vi "configAO_phi.vi"(7 "address":string, 8 "error in (no error)":errorcluster, 9 "new phi (deg)":dbl, 10 "AO Channel":i32, 11 "Channels: AO":T1={"AO amp (V)"=[0.01, 0.0, 0.0, 0.0, 0.0, 0.0, 0.0, 0.0], "AO DC (V)"=[0.0, 0.0, 0.0, 0.0, 0.0, 0.0, 0.0, 0.0], "AO f (Hz)"=[13.1, 13.0, 13.0, 13.0, 13.0, 13.0, 13.0, 13.0], "AO phi (deg)"=[0.0, 0.0, 0.0, 0.0, 0.0, 0.0, 0.0, 0.0], "function"=[enum."Sine Wave", enum."Sine Wave", enum."Sine Wave", enum."Sine Wave", enum."Sine Wave", enum."Sine Wave", enum."Sine Wave", enum."Sine Wave"]} {"AO f (Hz)" min=0.001 max=10000.0; "AO DC (V)" format="%#_6p"; "AO amp (V)" format="%#_6p"}) -> (0 "error out":errorcluster, 3 "Channels: AO":T1={"AO amp (V)"=[0.01, 0.0, 0.0, 0.0, 0.0, 0.0, 0.0, 0.0], "AO DC (V)"=[0.0, 0.0, 0.0, 0.0, 0.0, 0.0, 0.0, 0.0], "AO f (Hz)"=[13.1, 13.0, 13.0, 13.0, 13.0, 13.0, 13.0, 13.0], "AO phi (deg)"=[0.0, 0.0, 0.0, 0.0, 0.0, 0.0, 0.0, 0.0], "function"=[enum."Sine Wave", enum."Sine Wave", enum."Sine Wave", enum."Sine Wave", enum."Sine Wave", enum."Sine Wave", enum."Sine Wave", enum."Sine Wave"]} {"AO f (Hz)" min=0.001 max=10000.0; "AO DC (V)" format="%#_6p"; "AO amp (V)" format="%#_6p"})   [LabVIEW 2016]
doc: "API to configure an AO phase.\n\nSpecify which channel you want to change and the value you want to set.\n\nIf address=\"\", this API reads from localhost\nIf address is remote lockin, you need to add this computer to allowed whitelist on the lockin computer you are trying to access."
uses:
  Typedefs/AO-cluster.ctl
  Typedefs/AO_Amp-array.ctl
  Typedefs/AO_DC-array.ctl
  Typedefs/AO_f-array.ctl
  Typedefs/AO_phi-array.ctl
  Typedefs/Function-array.ctl
  Typedefs/Function-enum.ctl
panel:
  # "0"
  # "1"
  # "2"
  # "3"
  # "4"
  # "5"
  # "6"
  # "7"
  # "0"
  # "1"
  # "2"
  # "3"
  # "4"
  # "5"
  # "6"
  # "7"
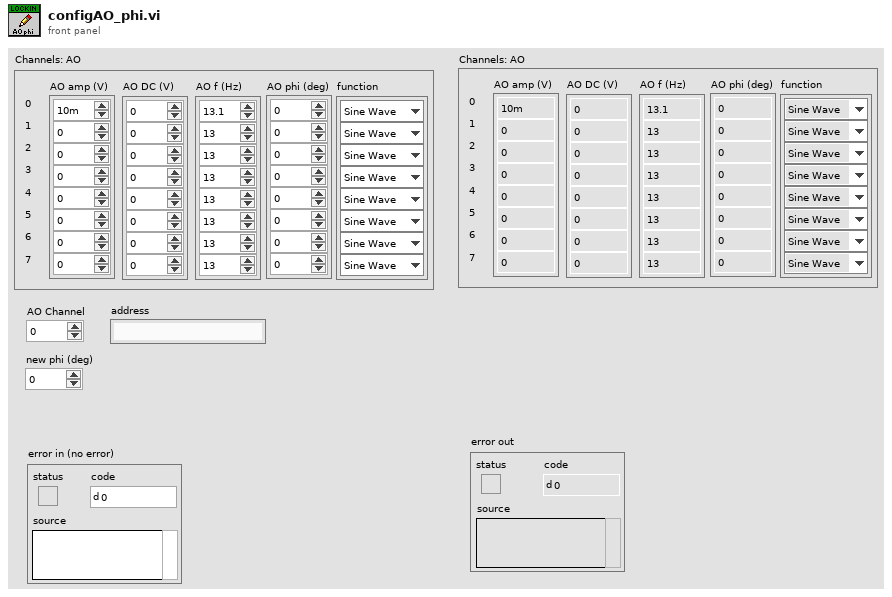
[diagram p1: front panel]
types:
  T1 = typedef "AO-cluster.ctl" = cluster{"AO amp (V)":T2, "AO DC (V)":T3, "AO f (Hz)":T4, "AO phi (deg)":T5, "function":T6}
  T2 = typedef "AO_Amp-array.ctl" = dbl[]
  T3 = typedef "AO_DC-array.ctl" = dbl[]
  T4 = typedef "AO_f-array.ctl" = dbl[]
  T5 = typedef "AO_phi-array.ctl" = dbl[]
  T6 = typedef "Function-array.ctl" = T7[]
  T7 = typedef "Function-enum.ctl" = enum16{"Sine Wave", "Triangle Wave", "Square Wave", "Sawtooth Wave"}
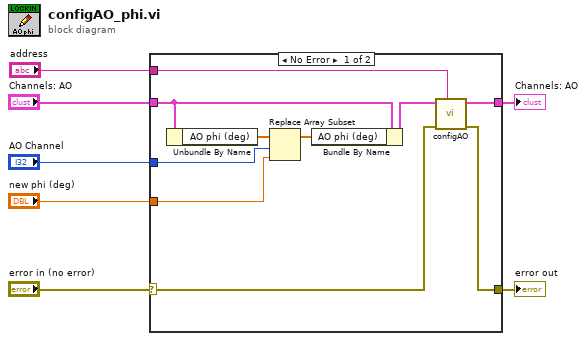
[diagram p0: block diagram]
diagram:
  n1 = case shown="No Error" "error in (no error)" {
    selector: "error in (no error)" -> [w10 w19]
    tunnel: "Channels: AO" -> [w15 w18]
    tunnel: [w11 w18] -> w6
    tunnel: "AO Channel" -> [w14 _]
    tunnel: "new phi (deg)" -> [w13 _]
    tunnel: [w9 w19] -> w2
    tunnel: "address" -> [w8 _]
    frame No Error {
      n2 = Unbundle By Name(w15) -> ("AO phi (deg)"=w16:T5)
      n3 = Replace Array Subset(array=w16, new element=w13, index=w14) -> (w17:T5)
      n4 = Bundle By Name(cluster=w15, "AO phi (deg)"=w17) -> (w12:T1)
      n5 = call "configAO.vi"("address"=w8, "error in (no error)"=w10, "Channels: AO in"=w12) -> ("error out"=w9:errorcluster, "Channels: AO out"=w11:T1)  [unwired: 7 in]
    }
    frame Error {
    }
  }
  "Channels: AO" <- w6
  "error out" <- w2
